vi "OutOfMemory-AnyThread.vi"(8 "No Error":errorcluster) -> (0 "error out":errorcluster)   [LabVIEW 2024, in "SDL3.lvlib" / "Error.lvlib"]
doc: "<B>LV Implementation Note</B>\nAs stated by the function doc, error strings are thread specific, that's why where are two OutOfMemory vi. One for UI Thread calls, the other for any thread.\n\n<B>Summary</B>\nSet an error indicating that memory allocation failed.\n\n<B>Remarks</B>\nThis function does not do any memory allocation."
uses:
  Error.lvlib
  Lib/SDL3-32.dll
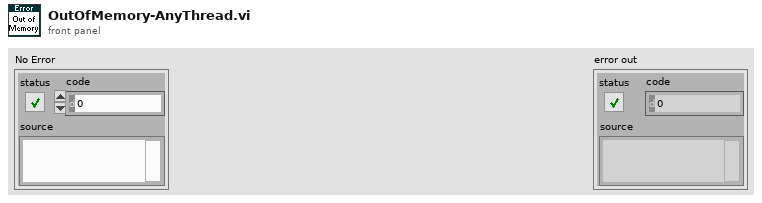
[diagram p1: front panel]
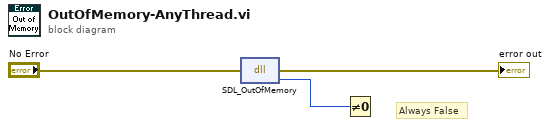
[diagram p0: block diagram]
diagram:
  # "Always False"
  n1 = dll-call lib="C:/Users/Thomas/Documents/Projects/LV-SDL3/Lib/SDL3-*.*" fn="SDL_OutOfMemory"(error in="No Error") -> (error out=→"error out":errorcluster, "return type"=w1:i32)  [unwired: 2 in, 1 out]
  n2 = Not Equal To 0?(x=w1) -> ()  [unwired: 1 out]
